vi "Motor_pwm.vi"() -> ()   [LabVIEW 2018]
uses:
  <vilib>/Waveform/WDTOps.llb/WDT Align Waveform Timestamps DBL.vi
panel:
  out "Erro":dbl
  out "x*y":dbl
  in  "Lambda/4":dbl(slide) scale=0.0..5.0
  in  "Controle da posição":dbl(knob) scale=-60.0..60.0
  out "Sentido":enum16{"Horário", "Anti-Horário"}(ring)
  in  "Tab Control":enum32{"Posição", "Velocidade", "Aceleração"}(tab)
  out "Posição Acumulada":waveform(dbl)(graph) caption="Velocidade"
  out "Velocidade Acumulada":waveform(dbl)[](graph) caption="Velocidade"
  out "Aceleração acumulada":waveform(dbl)(graph)
  out "Aceleração":dbl[](graph)
  out "Velocidade":dbl[][](graph)
  in  "Frequência do PWM":dbl
  in  "stop":bool
  out "Posição":dbl[](graph)
  in  "Initialize":bool
  in  "DC_Vin":dbl
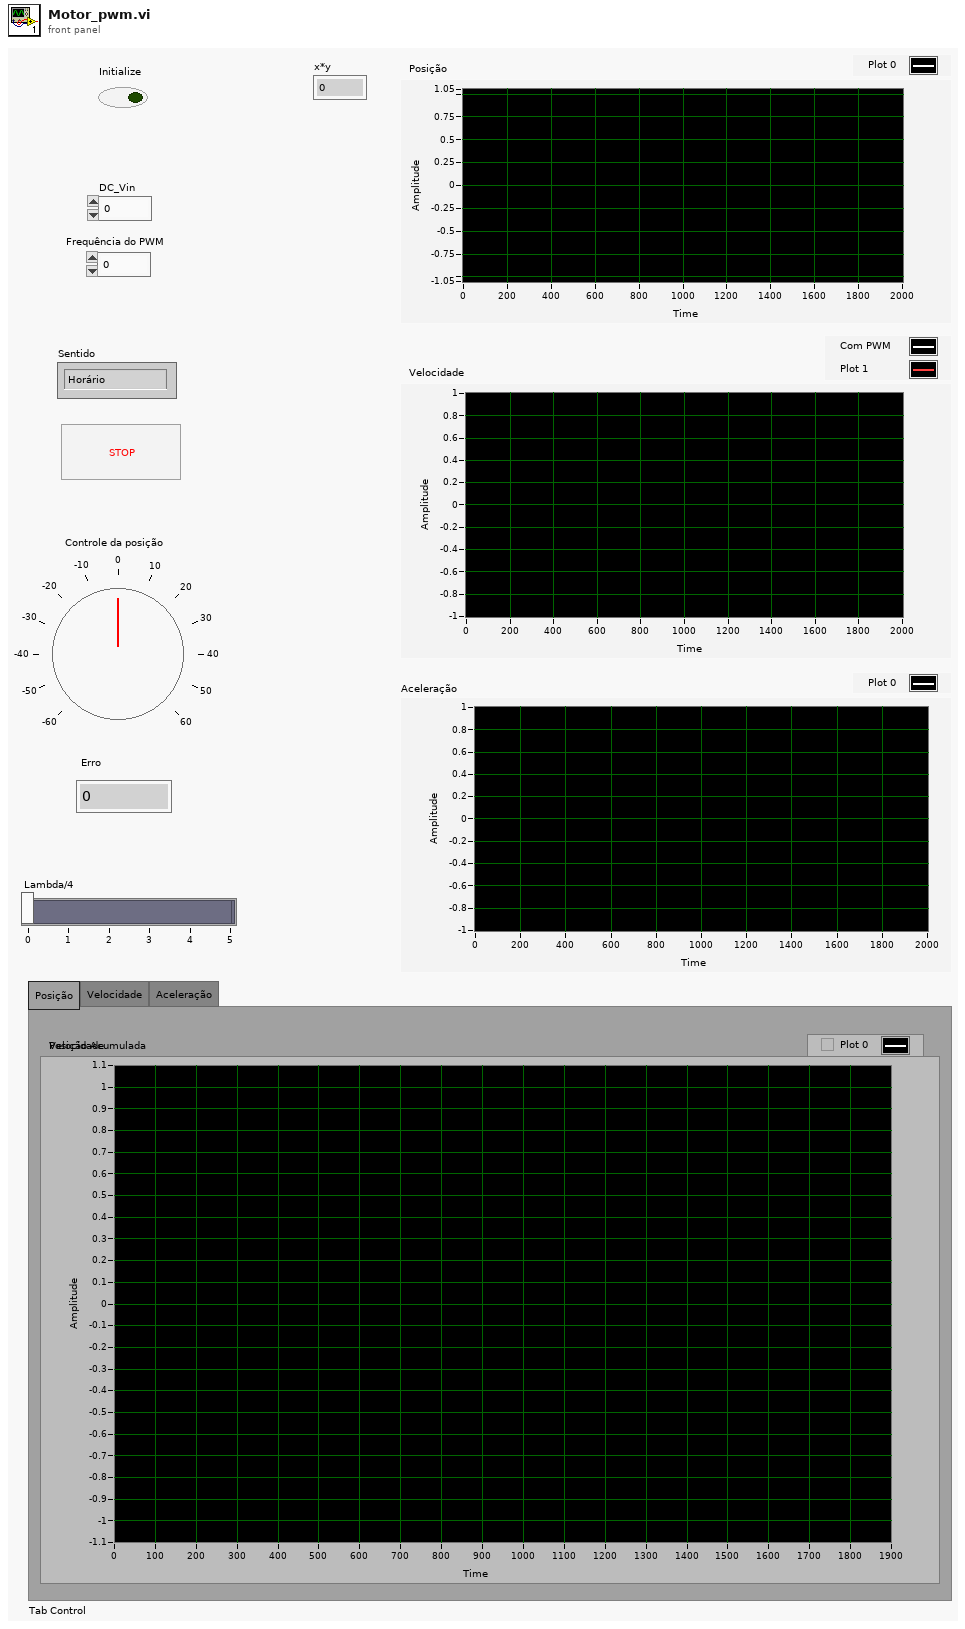
[diagram p1: front panel]
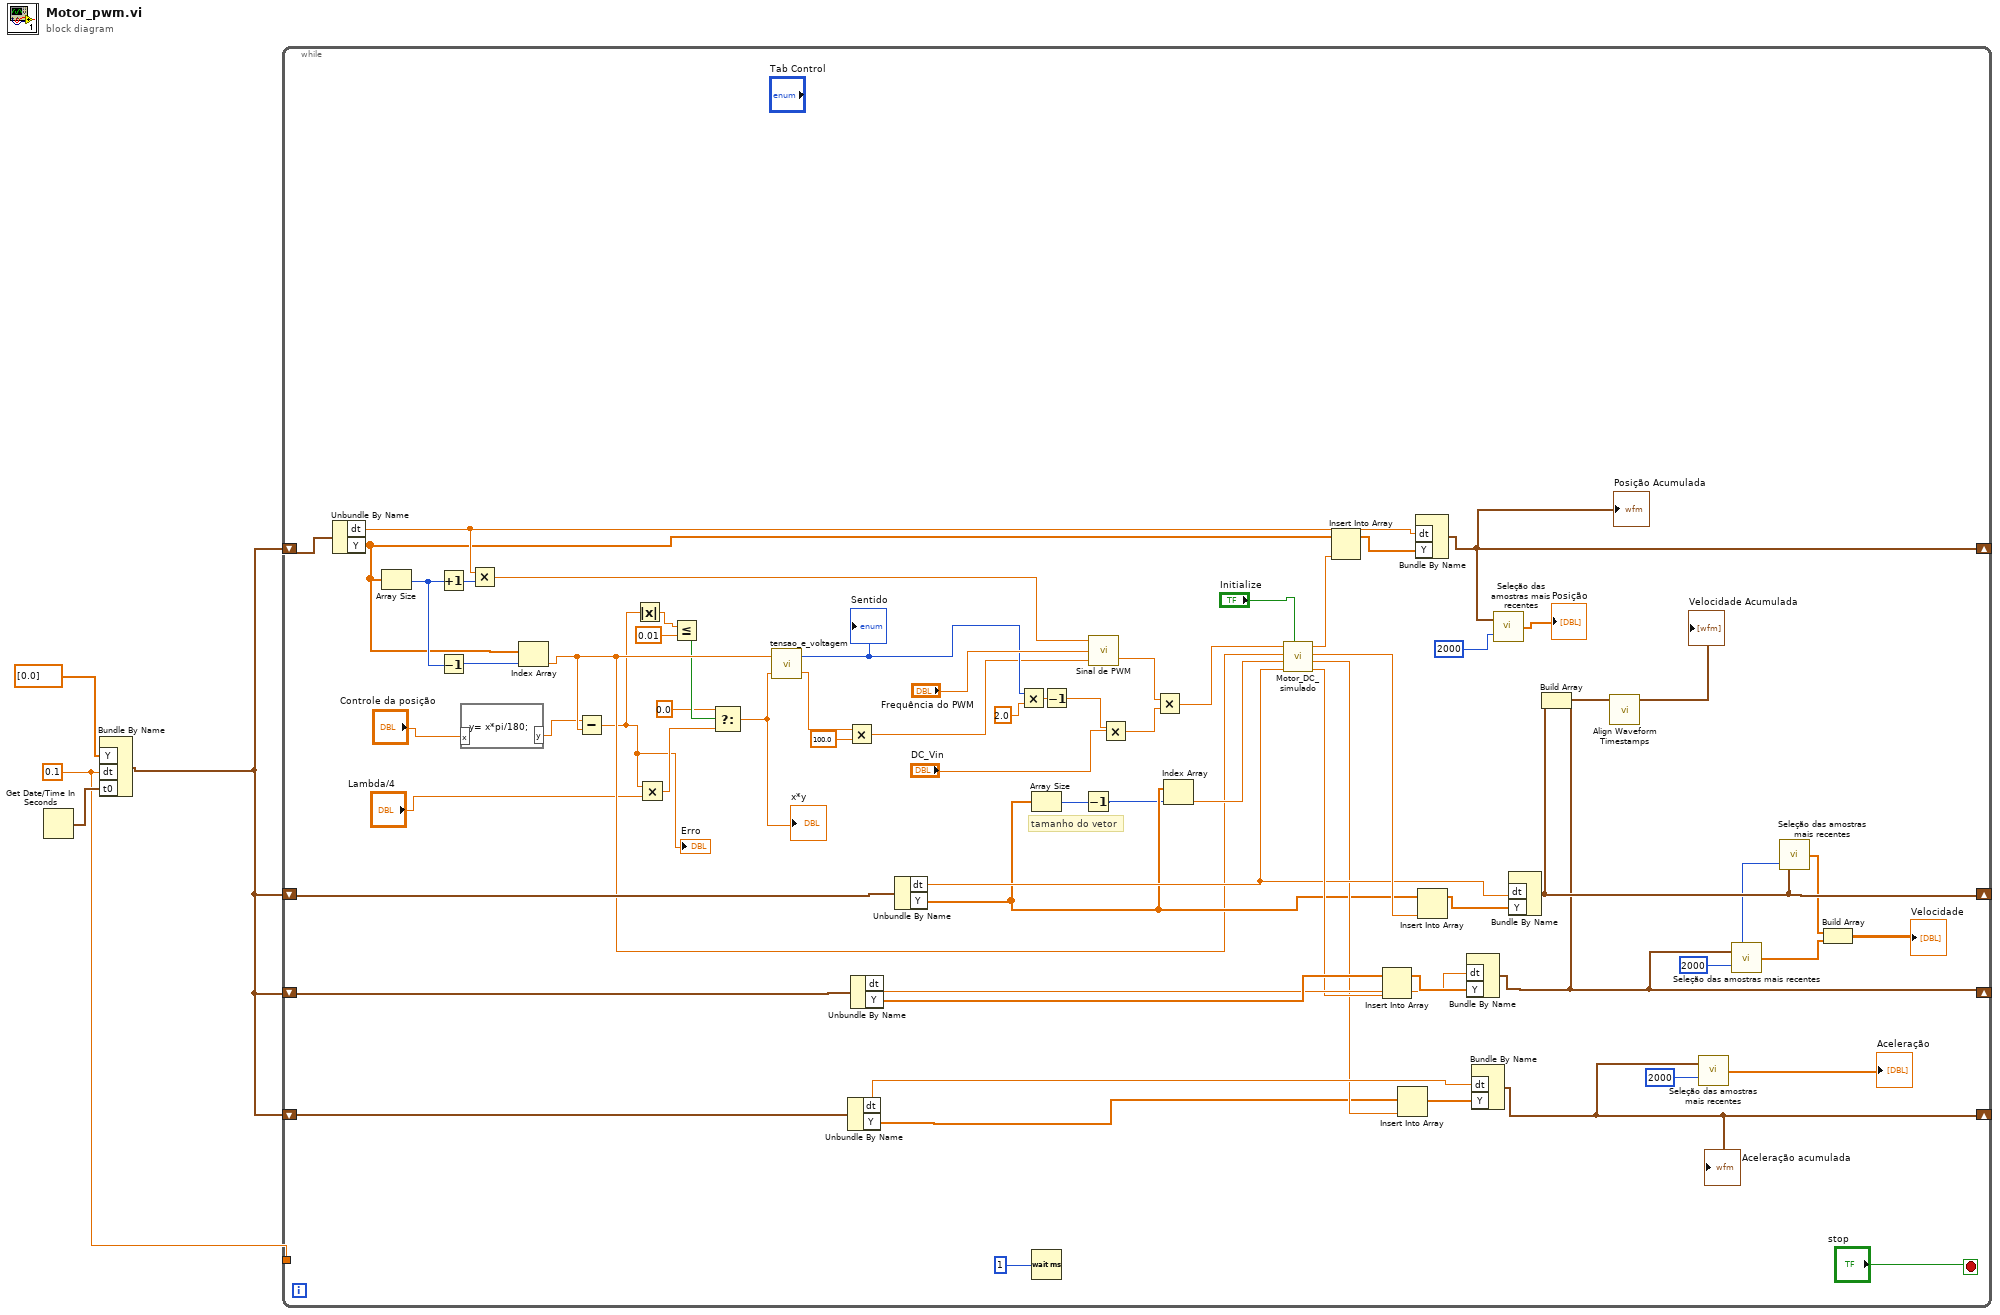
[diagram p0: block diagram]
diagram:
  w2 = 0.1 ("dt")
  n1 = Get Date/Time In Seconds() -> (seconds since 1Jan1904=w3:timestamp)
  n2 = Bundle By Name("Y"=dbl[] [0.0], "dt"=w2, "t0"=w3) -> (w1:waveform(dbl))  [unwired: 1 in]
  n3 = while {
    shift-right: [w51] -> _
    shift-left: w1 -> [w56]
    shift-right: [w50] -> _
    shift-left: w1 -> [w68]
    shift-right: [w49] -> _
    shift-left: w1 -> [w64]
    tunnel: w2 -> [_]
    shift-right: [w32] -> _
    shift-left: w1 -> [w35]
    stop <- "stop" stop-if-true
    w45 = 2000 ("Número de amostras no gráfico 2")
    # "tamanho do vetor"
    n4 = Unbundle By Name(w56) -> ("dt"=w26:dbl, "Y"=w23:dbl[])
    n5 = Array Size(array=w23) -> (size(s)=w24:i32)
    n6 = Increment(x=w24) -> (x+1=w55:i32)
    n7 = Decrement(x=w24) -> (x-1=w25:i32)
    n8 = formula code="y= x*pi/180;"("x"="Controle da posição") -> ("y"=w17:dbl)
    n9 = Multiply(x=w26, y=w55) -> (x*y=w21:dbl)
    n10 = Index Array(array=w23, index=w25) -> (element=w19:dbl)
    n11 = Subtract(x=w17, y=w19) -> (x-y=w5:dbl)
    "Erro" <- w5
    n12 = Absolute Value(x=w5) -> (abs(x)=w12:dbl)
    n13 = Multiply(x=w5, y="Lambda/4") -> (x*y=w8:dbl)
    n14 = Less Or Equal?(x=w12, y=0.01) -> (x <= y?=w9:bool)
    n15 = Select(t=0.0, s=w9, f=w8) -> (s? t:f=w6:dbl)
    "x*y" <- w6
    n16 = call "tensao_e_voltagem.vi"("T"=w6, "th"=w19) -> ("Duty Cycle"=w15:dbl, "Sentido"=w22:enum16{"Horário", "Anti-Horário"})
    "Sentido" <- w22
    n17 = Multiply(x=w15, y=100.0) -> (x*y=w13:dbl)
    n18 = Unbundle By Name(w35) -> ("dt"=w36:dbl, "Y"=w30:dbl[])
    n19 = Unbundle By Name(w64) -> ("dt"=w65:dbl, "Y"=w67:dbl[])
    n20 = Unbundle By Name(w68) -> ("dt"=w39:dbl, "Y"=w29:dbl[])
    n21 = Multiply(x=w22, y=2.0) -> (x*y=w43:dbl)
    n22 = Array Size(array=w29) -> (size(s)=w28:i32)
    n23 = Wait (ms)(milliseconds to wait=u32 1 ("y")) -> ()  [unwired: 1 out]
    n24 = Decrement(x=w43) -> (x-1=w41:dbl)
    n25 = Decrement(x=w28) -> (x-1=w27:i32)
    n26 = call "Sinal de PWM.vi"("duty cycle"=w13, "Frequência do PWM"="Frequência do PWM", "Tempo atual"=w21) -> ("Resultado numérico"=w58:dbl)  [unwired: 1 out]
    n27 = Multiply(x=w41, y="DC_Vin") -> (x*y=w40:dbl)
    n28 = Multiply(x=w58, y=w40) -> (x*y=w57:dbl)
    n29 = Index Array(array=w29, index=w27) -> (element=w38:dbl)
    n30 = call "Motor_DC_simulado.vi"("Initialize"="Initialize", "dt"=w39, "Velocidade anterior"=w38, "Posiçao anterior"=w19, "DC_Vin"=w57) -> ("Tensão fornecida ao motor"=w62:dbl, "Aceleração"=w34:dbl, "Velocidade"=w61:dbl, "Posição"=w60:dbl)  [unwired: 2 in]
    n31 = Insert Into Array(array=w23, new element=w60) -> (w70:dbl[])  [unwired: 1 in]
    n32 = Insert Into Array(array=w67, new element=w62) -> (w66:dbl[])  [unwired: 1 in]
    n33 = Insert Into Array(array=w30, new element=w34) -> (w37:dbl[])  [unwired: 1 in]
    n34 = Bundle By Name("dt"=w26, "Y"=w70) -> (w51:waveform(dbl))  [unwired: 1 in]
    "Posição Acumulada" <- w51
    n35 = Insert Into Array(array=w29, new element=w61) -> (w69:dbl[])  [unwired: 1 in]
    n36 = Bundle By Name("dt"=w65, "Y"=w66) -> (w49:waveform(dbl))  [unwired: 1 in]
    n37 = Bundle By Name("dt"=w36, "Y"=w37) -> (w32:waveform(dbl))  [unwired: 1 in]
    "Aceleração acumulada" <- w32
    n38 = call "Seleção das amostras mais recentes.vi"("Número de amostras no gráfico"=2000, "Vetor de entrada"=w51) -> ("Amostras do gráfico"=→"Posição":dbl[])
    n39 = Bundle By Name("dt"=w39, "Y"=w69) -> (w50:waveform(dbl))  [unwired: 1 in]
    n40 = Build Array "Build Array"(w50, w49) -> (w63:waveform(dbl)[])
    n41 = call-poly <vilib>:"Align Waveform Timestamps.vi"("waveforms in"=w63) -> ("waveforms out"=→"Velocidade Acumulada":waveform(dbl)[])  [unwired: 9 in, 1 out]
    n42 = call "Seleção das amostras mais recentes.vi"("Número de amostras no gráfico"=2000 ("Número de amostras no gráfico 2"), "Vetor de entrada"=w32) -> ("Amostras do gráfico"=→"Aceleração":dbl[])
    n43 = call "Seleção das amostras mais recentes.vi"("Número de amostras no gráfico"=w45, "Vetor de entrada"=w49) -> ("Amostras do gráfico"=w48:dbl[])
    n44 = call "Seleção das amostras mais recentes.vi"("Número de amostras no gráfico"=w45, "Vetor de entrada"=w50) -> ("Amostras do gráfico"=w47:dbl[])
    n45 = Build Array "Build Array"(w47, w48) -> (→"Velocidade":dbl[][])
  }
